vi "CAL-Load data V1.vi"(0 "user path":path, 11 "error in (no error)":errorcluster) -> (4 "new file path":path, 6 "Frequency":dbl[](array[numeric]), 8 "Mag":dbl[](array[numeric]), 10 "Phase":dbl[](array[numeric]), 13 "npts":i32, 14 "Fs (Hz)":dbl, 15 "error out":errorcluster)   [LabVIEW 2020]
uses:
  <vilib>/Utility/file.llb/Read From Spreadsheet File (DBL).vi
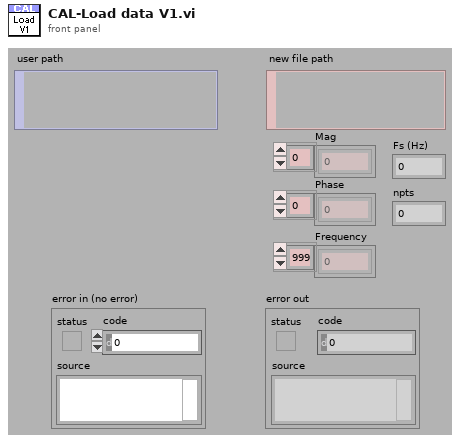
[diagram p1: front panel]
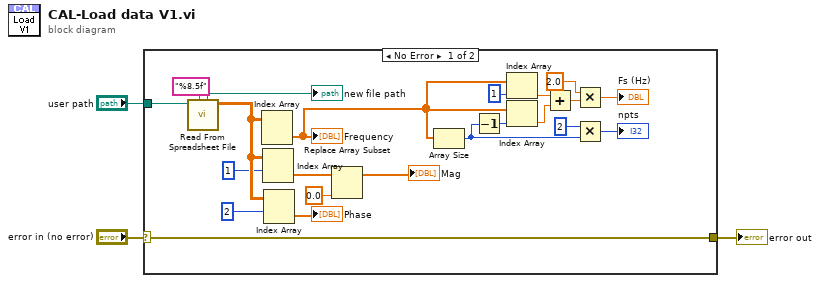
[diagram p0: block diagram]
diagram:
  n1 = case shown="No Error" "error in (no error)" {
    selector: "error in (no error)" -> [w4 w26]
    tunnel: "user path" -> [w5 _]
    tunnel: [w4 w26] -> w2
    frame No Error {
      n2 = call-poly <vilib>:"Read From Spreadsheet File.vi"("format (%.3f)"="%8.5f", "file path (dialog if empty)"=w5) -> ("all rows"=w23:dbl[][], "new file path (Not A Path if cancelled)"=→"new file path":path)  [unwired: 5 in, 3 out]
      n3 = Index Array(array=w23) -> (element=w11:dbl[])  [unwired: 2 in]
      "Frequency" <- w11
      n4 = Index Array(array=w23, index (row)=1) -> (element=w8:dbl[])  [unwired: 1 in]
      n5 = Index Array(array=w23, index (row)=2) -> (element=→"Phase":dbl[])  [unwired: 1 in]
      n6 = Replace Array Subset(array=w8, new element=0.0 ("new element/subarray")) -> (→"Mag":dbl[])  [unwired: 1 in]
      n7 = Array Size(array=w11) -> (size(s)=w18:i32)
      n8 = Decrement(x=w18) -> (x-1=w19:i32)
      n9 = Index Array(array=w11, index=1) -> (element=w14:dbl)
      n10 = Index Array(array=w11, index=w19) -> (element=w13:dbl)
      n11 = Add(x=w14, y=w13) -> (x+y=w15:dbl)
      n12 = Multiply(x=2.0, y=w15) -> (x*y=→"Fs (Hz)":dbl)
      n13 = Multiply(x=2, y=w18) -> (x*y=→"npts":i32)
    }
    frame Error {
    }
  }
  "error out" <- w2
